vi "Step_Selection.vi"(10 "Current position":u16, 11 "Desired position":u16) -> (3 "Step":u16)   [LabVIEW 2015]
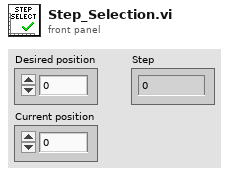
[diagram p1: front panel]
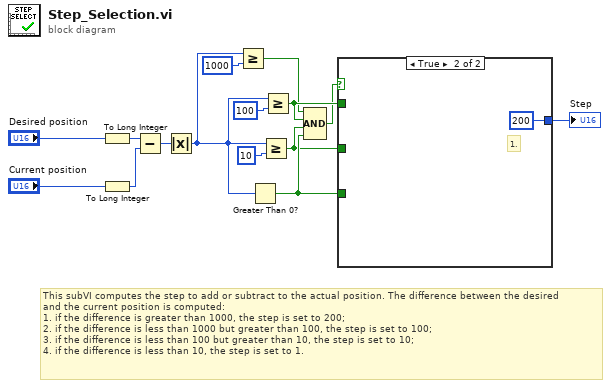
[diagram p0: block diagram]
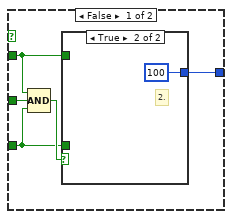
[diagram p2: hidden frame]
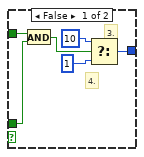
[diagram p3: hidden frame]
diagram:
  # "This subVI computes the step to add or subtract to the actual position. The difference between the desired\nand the current position is computed:\n1. if the difference is greater than 1000, the step is set to 200;\n2. if the difference is less than 1000 but greater than 100, the step is set to 100;\n3. if the difference is less than 100 but greater than 10, the step is set to 10;\n4. if the difference is less than 10, the step is set to 1."
  n1 = To Long Integer(number="Desired position") -> (32bit integer=w4:i32)
  n2 = To Long Integer(number="Current position") -> (32bit integer=w5:i32)
  n3 = Subtract(x=w4, y=w5) -> (x-y=w2:i32)
  n4 = Absolute Value(x=w2) -> (abs(x)=w11:i32)
  n5 = Greater Or Equal?(x=w11, y=1000) -> (x >= y?=w9:bool)
  n6 = Greater Than 0?(x=w11) -> (x > 0?=w15:bool)
  n7 = Greater Or Equal?(x=w11, y=10) -> (x >= y?=w14:bool)
  n8 = Greater Or Equal?(x=w11, y=100) -> (x >= y?=w13:bool)
  n9 = Compound Arithmetic op=AND(w9, w13, w14, w15) -> (w12:bool)
  n10 = case shown="True" w12 {
    tunnel: [w18 u16 200 ("y")] -> w1
    tunnel: w13 -> [w17 _]
    tunnel: w14 -> [w20 _]
    tunnel: w15 -> [w16 _]
    frame False {
      n11 = Compound Arithmetic op=AND(w17, w20, w16) -> (w19:bool)
      n12 = case shown="True" w19 {
        tunnel: [w21 u16 100 ("y")] -> w18
        tunnel: w17 -> [w26 _]
        tunnel: w16 -> [w25 _]
        frame False {
          # "3."
          # "4."
          n13 = And(x=w26, y=w25) -> (x .and. y?=w24:bool)
          n14 = Select(t=u16 10 ("y"), s=w24, f=u16 1) -> (s? t:f=w21:u16)
        }
        frame True {
          # "2."
        }
      }
    }
    frame True {
      # "1."
    }
  }
  "Step" <- w1
